vi "TimeTable_Head.vi"(2 "input file":refnum<file>, 3 "error in":errorcluster) -> (0 "output file refnum":refnum<file>, 1 "error out":errorcluster)   [LabVIEW 2018]
doc: "Подприбор вставляет в шапку таблицы (txt-файла) надписи Time и World Time"
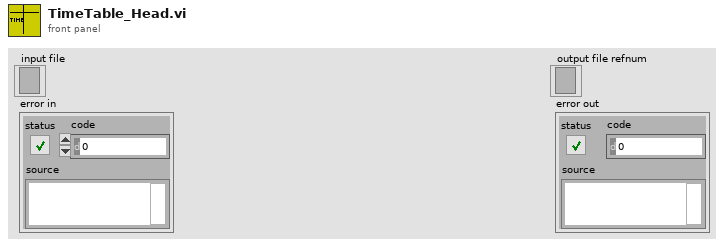
[diagram p1: front panel]
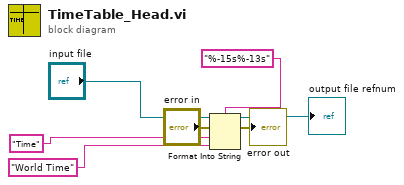
[diagram p0: block diagram]
diagram:
  n1 = Format Into String(format string="%-15s%-13s", initial string="input file", error in="error in", "Time" ("text"), "World Time") -> (resulting string=→"output file refnum":refnum<file>, error out=→"error out":errorcluster)
